vi "Serialize.vi"(8 "error in (no error)":errorcluster, 11 "SubVIConverter in":refnum<class "SubVIConverter.lvclass">) -> (0 "error out":errorcluster, 2 "JSON":string, 3 "SubVIConverter out":refnum<class "SubVIConverter.lvclass">)   [LabVIEW 2017, in "SubVIConverter.lvclass"]
uses:
  SubVIConverter.lvclass
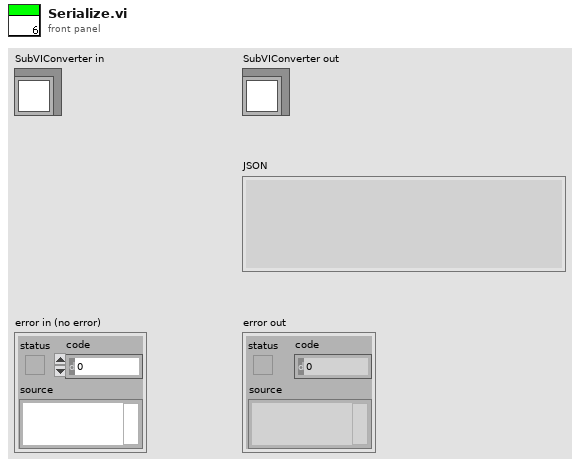
[diagram p1: front panel]
types:
  T1 = typedef "LVRectTypeDef.ctl" = cluster{"Left":i16, "Top":i16, "Right":i16, "Bottom":i16}
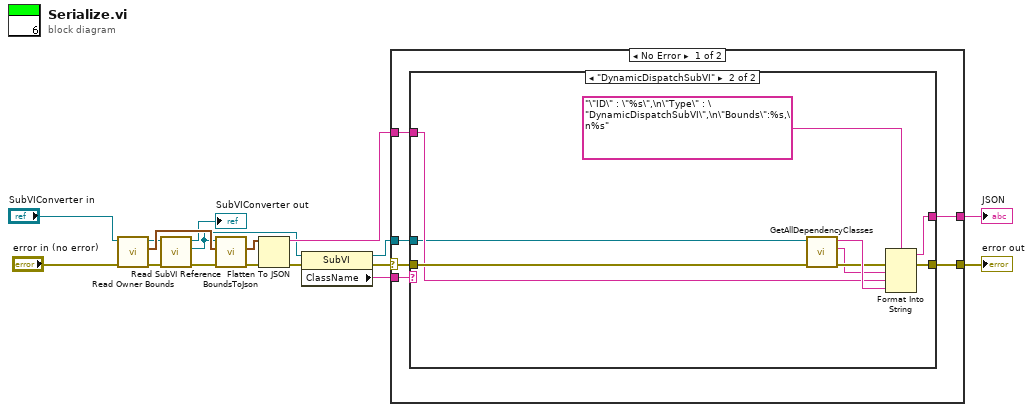
[diagram p0: block diagram]
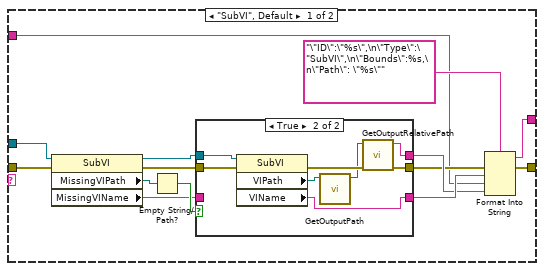
[diagram p2: hidden frame]
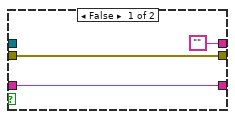
[diagram p3: hidden frame]
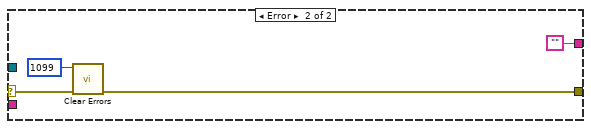
[diagram p4: hidden frame]
diagram:
  n1 = call-dynamic "Read Owner Bounds.vi"("error in (no error)"="error in (no error)", "VIObjectConverter in"="SubVIConverter in") -> ("error out"=w5:errorcluster, "Rect"=w16:T1, "VIObjectConverter out"=w7:refnum<class "SubVIConverter.lvclass">)  [unwired: 7 in]
  n2 = call-dynamic "Read SubVI Reference.vi"("error in (no error)"=w5, "SubVIConverter in"=w7) -> ("error out"=w4:errorcluster, "SubVI Reference"=w2:refnum<vi>, "SubVIConverter out"=→"SubVIConverter out":refnum<class "SubVIConverter.lvclass">)  [unwired: 7 in]
  n3 = call "BoundsToJson.vi"("error in (no error)"=w4, "Owner Bounds"=w16, "GObj in"=w2) -> ("error out"=w9:errorcluster, "Relative Bounds"=w10:cluster{"x":i32, "y":i32, "w":i32, "h":i32})  [unwired: 5 in, 2 out]
  n4 = Flatten To JSON(anything=w10, error in (no error)=w9) -> (JSON string=w14:string, 11:w12:errorcluster)  [unwired: 1 in]
  n5 = property class="SubVI"(reference=w2, error in=w12) -> (reference out=w1:refnum<vi>, error out=w11:errorcluster, "ClassName"=w13:string)
  n6 = case shown="No Error" w11 {
    selector: w11 -> [w18 w58]
    tunnel: w14 -> [w23 _]
    tunnel: w13 -> [w22 _]
    tunnel: w1 -> [w21 _]
    tunnel: [w20 ""] -> w8
    tunnel: [w19 w61] -> w3
    frame No Error {
      n7 = case shown="\"DynamicDispatchSubVI\"" w22 {
        tunnel: w21 -> [w28 w51]
        tunnel: w18 -> [w27 w57]
        tunnel: [w24 w55] -> w19
        tunnel: [w25 w54] -> w20
        tunnel: w23 -> [w26 w52]
        frame "SubVI", Default {
          n8 = property class="SubVI"(reference=w28, error in=w27) -> (reference out=w34:refnum<vi>, error out=w33:errorcluster, "MissingVIPath"=w37:path, "MissingVIName"=w35:string)
          n9 = Empty String/Path?(string/path=w37) -> (empty?=w36:bool)
          n10 = case shown="True" w36 {
            tunnel: ["" w45] -> w30
            tunnel: [w40 w48] -> w31
            tunnel: w35 -> [w40 _]
            tunnel: w34 -> [_ w47]
            tunnel: w33 -> [w39 w46]
            tunnel: [w39 w43] -> w29
            frame False {
            }
            frame True {
              n11 = property class="SubVI"(reference=w47, error in=w46) -> (error out=w44:errorcluster, "VIPath"=w42:path, "VIName"=w48:string)  [unwired: 1 out]
              n12 = call "GetOutputPath.vi"("Path"=w42) -> ("Output Path"=w41:path)  [unwired: 10 in]
              n13 = call "GetOutputRelativePath.vi"("error in (no error)"=w44, "Path"=w41) -> ("error out"=w43:errorcluster, "Output relative path"=w45:string)  [unwired: 8 in]
            }
          }
          n14 = Format Into String(format string="\"ID\":\"%s\",\n\"Type\":\"SubVI\",\n\"Bounds\":%s,\n\"Path\": \"%s\"", error in=w29, w31, w26, w30) -> (resulting string=w25:string, error out=w24:errorcluster)  [unwired: 1 in]
        }
        frame "DynamicDispatchSubVI" {
          n15 = call "GetAllDependencyClasses.vi"("error in (no error)"=w57, "SubVI in"=w51) -> ("error out"=w50:errorcluster, "VI Name"=w49:string, "Implementations JSON string"=w56:string)  [unwired: 7 in]
          n16 = Format Into String(format string="\"ID\" : \"%s\",\n\"Type\" : \"DynamicDispatchSubVI\",\n\"Bounds\":%s,\n%s", error in=w50, w49, w52, w56) -> (resulting string=w54:string, error out=w55:errorcluster)  [unwired: 1 in]
        }
      }
    }
    frame Error {
      n17 = call <vilib>:"Clear Errors.vi"("error in (no error)"=w58, "specific error code to clear (0: all)"=1099) -> ("error out"=w61:errorcluster)  [unwired: 4 in, 1 out]
    }
  }
  "error out" <- w3
  "JSON" <- w8
